vi "ClearReference.vi"(1 "reference in":refnum<class "G#RemoteProxy.lvclass">) -> (0 "reference out":refnum<class "G#RemoteProxy.lvclass">)   [LabVIEW 2017, in "G#RemoteProxy.lvclass"]
doc: "Clears the object reference and makes it invalid.\n\nNotice, this will not delete the object!"
uses:
  <vilib>/addons/_AddQ/G#Debugger/G#RemoteProxy/G#RemoteProxy.lvclass
  <vilib>/addons/_AddQ/G#Debugger/G#RemoteProxy/G#RemoteProxy.lvclass/G#RemoteProxy.ctl
  <vilib>/addons/_AddQ/G#Object/G#Object.lvclass
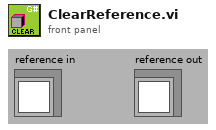
[diagram p1: front panel]
types:
  T1 = typedef "G#RemoteProxy.lvclass/ObjectAttributesProxy.ctl" = cluster{"class hierarchy":T2[], "class name":string, "lvlib hierarchy":string[], "full class name":string, "id":u32, "owner":string, "RemoteRef":refnum<class "G#Object.lvclass">, "object name":string, "attributes":variant[], "connection ID":refnum<k5>, "address":u32, "occurrence":refnum<k4>, "ProxyClassRef":refnum<class "G#RemoteProxy.lvclass">, "InMemory?":bool, "ToString":string}
  T2 = typedef "G#Object.lvclass/G#Object_ClassHierarchy.ctl" = cluster{"ClassName":string, "FullClassName":string, "ClassPath":path, "IsLeaf":bool}
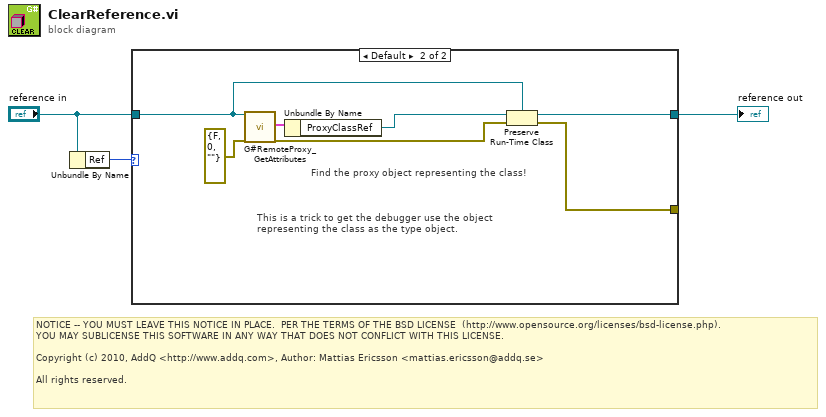
[diagram p0: block diagram]
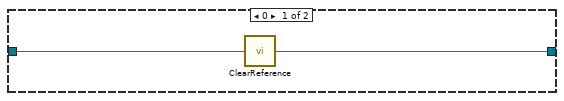
[diagram p2: hidden frame]
diagram:
  # "NOTICE -- YOU MUST LEAVE THIS NOTICE IN PLACE.  PER THE TERMS OF THE BSD LICENSE  (http://www.opensource.org/licenses/bsd-license.php).\nYOU MAY SUBLICENSE THIS SOFTWARE IN ANY WAY THAT DOES NOT CONFLICT WITH THIS LICENSE.\n\nCopyright (c) 2010, AddQ <http://www.addq.com>, Author: Mattias Ericsson <mattias.ericsson@addq.se>\n\nAll rights reserved."
  n1 = Unbundle By Name("reference in") -> ("Ref"=w3:u32)
  n2 = case shown="Default" w3 {
    tunnel: "reference in" -> [w5 w10]
    tunnel: [w4 w9] -> w1
    tunnel: [_ w7] -> _
    frame 0 {
      n3 = call-parent "ClearReference.vi"("reference in"=w5) -> ("reference out"=w4:refnum<class "G#RemoteProxy.lvclass">)
    }
    frame Default {
      # "This is a trick to get the debugger use the object\nrepresenting the class as the type object."
      # "Find the proxy object representing the class!"
      n4 = call <vilib>:"G#RemoteProxy_GetAttributes.vi"("reference in"=w10, "error in (no error)"=errorcluster {"status"=FALSE, "code"=0, "source"=""}) -> ("attributes"=w11:T1, "error out"=w8:errorcluster)  [unwired: 14 in, 2 out]
      n5 = Unbundle By Name(w11) -> ("ProxyClassRef"=w6:refnum<class "G#RemoteProxy.lvclass">)
      n6 = Preserve Run-Time Class(object in=w6, error in=w8, 2:w10) -> (object out=w9:refnum<class "G#RemoteProxy.lvclass">, error out=w7:errorcluster)
    }
  }
  "reference out" <- w1
